vi "rad_IPaddr and Password Global.vi"(7 "Read(F)/Write(T)":bool, 10 "Password":string, 11 "IP/MAC Address":string) -> (2 "Password":string, 3 "IP/MAC Address":string)   [LabVIEW 2020]
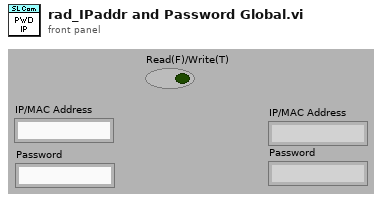
[diagram p1: front panel]
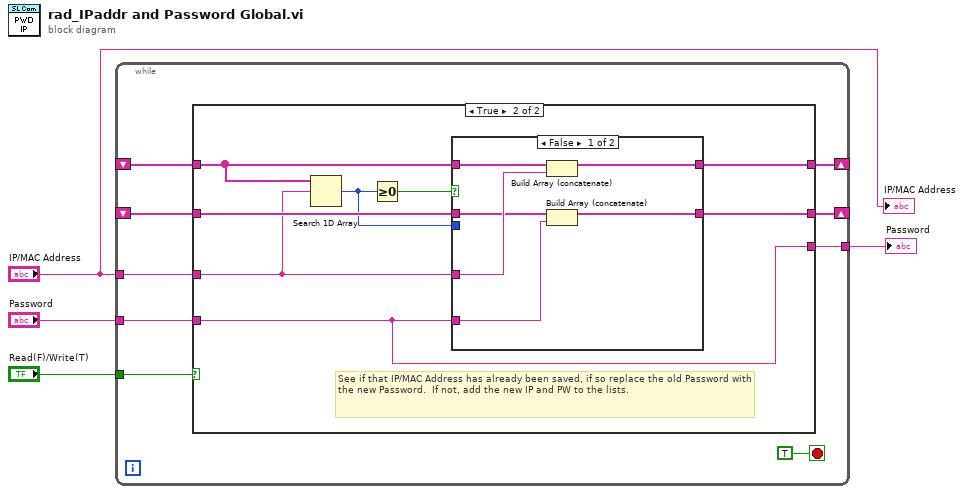
[diagram p0: block diagram]
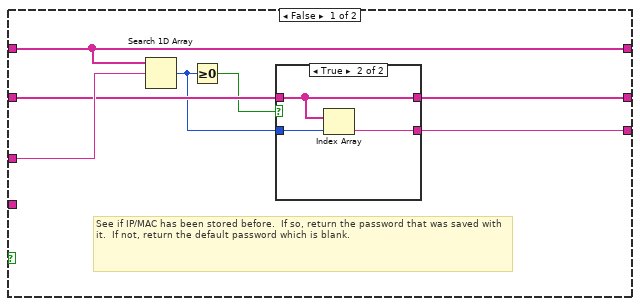
[diagram p2: hidden frame]
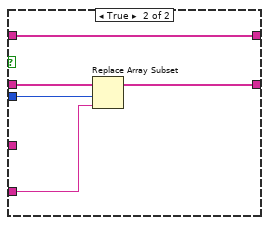
[diagram p4: hidden frame]
diagram:
  n1 = while {
    shift-right: [w6] -> _
    shift-left: _ -> [w9]
    tunnel: "Read(F)/Write(T)" -> [w12]
    tunnel: "IP/MAC Address" -> [w11]
    tunnel: "Password" -> [w10]
    shift-right: [w7] -> _
    shift-left: _ -> [w8]
    tunnel: [w5] -> w2
    stop <- TRUE stop-if-true
    n2 = case shown="True" w12 {
      tunnel: w11 -> [w19 w26]
      tunnel: w10 -> [_ w25]
      tunnel: w9 -> [w20 w29]
      tunnel: w8 -> [w18 w31]
      tunnel: [w16 w30] -> w7
      tunnel: [w20 w27] -> w6
      tunnel: [w14 w25] -> w5
      frame False {
        # "See if IP/MAC has been stored before.  If so, return the password that was saved with it.  If not, return the default password which is blank."
        n3 = Search 1D Array(1D array=w20, element=w19) -> (index of element=w15:i32)  [unwired: 1 in]
        n4 = Greater Or Equal To 0?(x=w15) -> (x >= 0?=w17:bool)
        n5 = case shown="True" w17 {
          tunnel: w18 -> [w21 w24]
          tunnel: [w21 w24] -> w16
          tunnel: w15 -> [_ w23]
          tunnel: [_ w22] -> w14
          frame False {
          }
          frame True {
            n6 = Index Array(array=w24, index=w23) -> (element=w22:string)
          }
        }
      }
      frame True {
        # "See if that IP/MAC Address has already been saved, if so replace the old Password with the new Password.  If not, add the new IP and PW to the lists."
        n7 = Search 1D Array(1D array=w29, element=w26) -> (index of element=w28:i32)  [unwired: 1 in]
        n8 = Greater Or Equal To 0?(x=w28) -> (x >= 0?=w32:bool)
        n9 = case shown="False" w32 {
          tunnel: w31 -> [w35 w43]
          tunnel: [w34 w42] -> w30
          tunnel: w29 -> [w38 w39]
          tunnel: w28 -> [_ w41]
          tunnel: w25 -> [w33 w40]
          tunnel: [w37 w39] -> w27
          tunnel: w26 -> [w36 _]
          frame False {
            n10 = Build Array (concatenate)(w38, w36) -> (w37:string[])
            n11 = Build Array (concatenate)(w35, w33) -> (w34:string[])
          }
          frame True {
            n12 = Replace Array Subset(array=w43, new element=w40, index=w41) -> (w42:string[])
          }
        }
      }
    }
  }
  "Password" <- w2
  "IP/MAC Address" <- "IP/MAC Address"
